vi "Prepare Scan Data to Array.vi"(10 "Distance":u32[](array[numeric]) format="%08x", 11 "Packet A":T1 {"Scan Number" format="%04d"; "Status Flags" format="%04x"; "Timestamp Sync" format="%016x"; "Timestamp Raw" format="%016x"; "Packet Number" format="%04d"; "Header Size" format="%04d"; "Packet Size" format="%04x"; "Packet Type" format="%04x"}) -> (3 "Distance x Angle":cluster{"Magnitude":dbl, "Phase":dbl}[](array[cluster]))   [LabVIEW 2019, in "PF_API.lvclass"]
uses:
  PF_API.lvclass
  Packet Structure A.ctl
panel:
  out "Array":cluster{dbl, dbl}[](array[cluster])
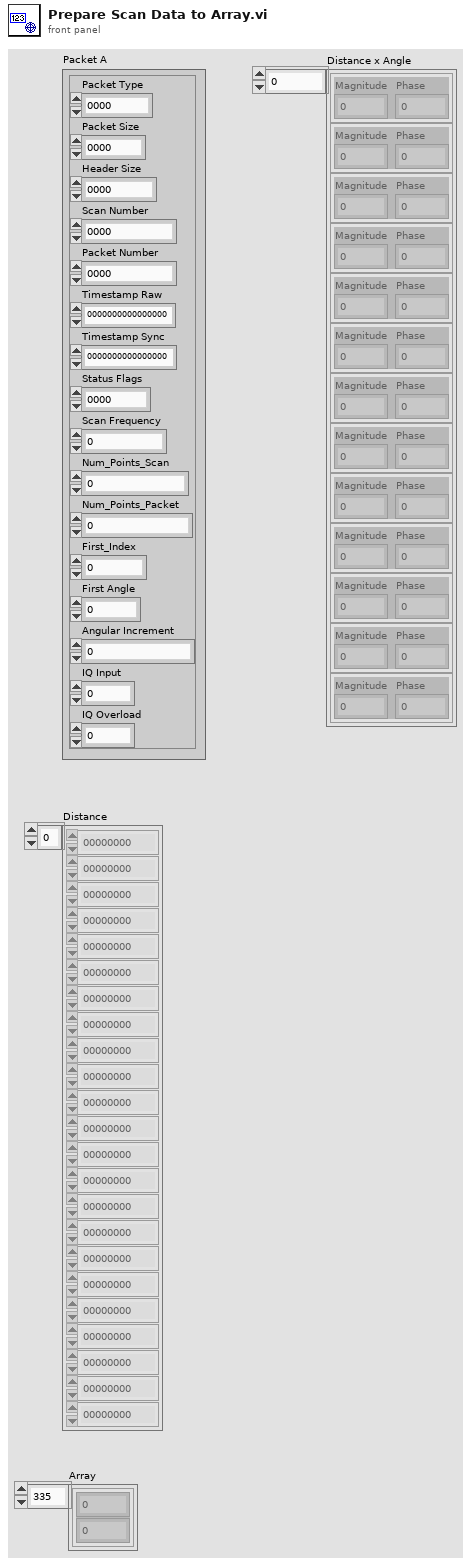
[diagram p1: front panel]
types:
  T1 = typedef "PF_API.lvclass/Packet Structure A.ctl" = cluster{"Packet Type":u16, "Packet Size":u32, "Header Size":u16, "Scan Number":u16, "Packet Number":u16, "Timestamp Raw":u64, "Timestamp Sync":u64, "Status Flags":u32, "Scan Frequency":u32, "Num_Points_Scan":u16, "Num_Points_Packet":u16, "First_Index":u16, "First Angle":i32, "Angular Increment":i32, "IQ Input":u32, "IQ Overload":u32}
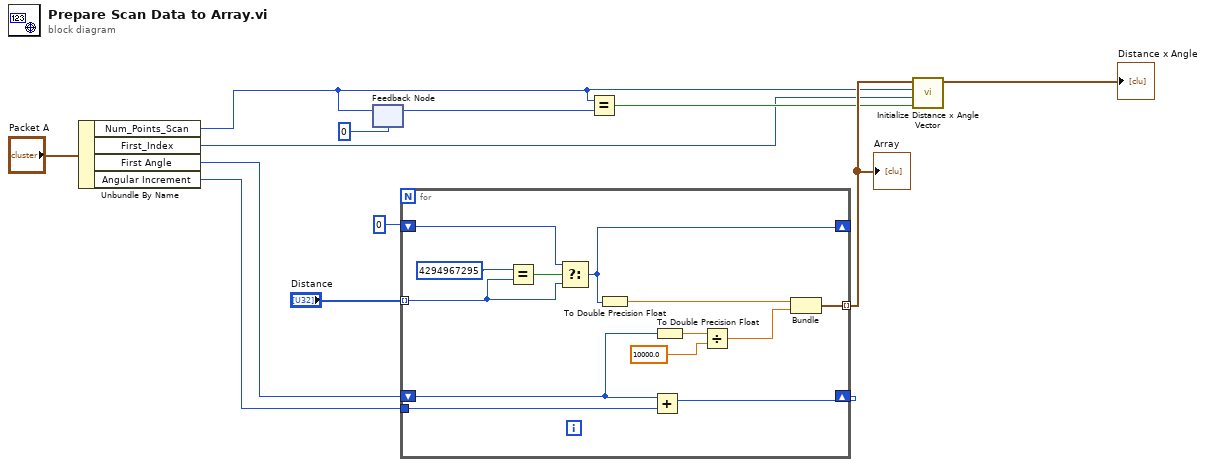
[diagram p0: block diagram]
diagram:
  n1 = Unbundle By Name("Packet A") -> ("Num_Points_Scan"=w3:u16, "First_Index"=w2:u16, "First Angle"=w8:i32, "Angular Increment"=w7:i32)
  n2 = feedback-in #1(w3) -> ()
  n3 = feedback #1(u16 0 ("Num_Points_Scan")) -> (w10:u16)
  n4 = for {
    tunnel: "Distance" -> [w14] mode=indexing
    tunnel: w7 -> [w25]
    shift-right: [w24] -> _
    shift-left: w8 -> [w22]
    tunnel: [w18] -> w5 mode=indexing
    shift-right: [w13] -> _
    shift-left: 0 -> [w15]
    n5 = Equal?(x=u32 4294967295, y=w14) -> (x = y?=w16:bool)
    n6 = Select(t=w15, s=w16, f=w14) -> (s? t:f=w13:u32)
    n7 = To Double Precision Float(number=w13) -> (double precision float=w20:dbl)
    n8 = Add(x=w22, y=w25) -> (x+y=w24:i32)
    n9 = To Double Precision Float(number=w22) -> (double precision float=w23:dbl)
    n10 = Divide(x=w23, y=10000.0) -> (x/y=w19:dbl)
    n11 = Bundle(w20, w19) -> (w18:cluster{dbl, dbl})  [unwired: 1 in]
  }
  "Array" <- w5
  n12 = Equal?(x=w3, y=w10) -> (x = y?=w4:bool)
  n13 = call "Initialize Distance x Angle Vector.vi"("Boolean"=w4, "First Index"=w2, "Num_Points_Scan"=w3, "Distance x Angle In"=w5) -> ("Distance x Angule"=→"Distance x Angle":cluster{"Magnitude":dbl, "Phase":dbl}[])  [unwired: 7 in]
